vi "fpgaAcquire_exttrigtest.vi"(0 "Trigger address":i16=1500, 1 "Command FIFO":refnum<k21>, 2 "Circular Buffer Mem":refnum<k21>, 3 "circular buffer length":u32=300, 5 "Fake data in":i16, 6 "Timing FIFO":refnum<k21>, 7 "channel on/off":bool, 9 "Trigger":i16=1500, 11 "Samples to Acquire":u32=95, 12 "Is Test Pulse?":bool, 13 "# of pretrigger":u32=15, 14 "timing":u64) -> ()   [LabVIEW 2012]
uses:
  <vilib>/rvi/DataTransferAndStorage/Container/Common/niFpgaContainerExecOnDevCompGetState.vi
  <vilib>/rvi/Emulation/niFpgaSctlEmulationGetInTimedLoop.vi
  <vilib>/rvi/DataTransferAndStorage/Container/Common/niFpgaContainerGetUniqueNameForEmu.vi
  <vilib>/rvi/FIFO/Fifo_Resource/nirvififoEmulationSetSize.vi
  <vilib>/rvi/errors/niFpgaSetErrorForExecOnDevCompSimple.vi
  <vilib>/rvi/eio/common/nirviEmuReportErrorAndStop.vi
  <vilib>/rvi/Emulation/niFpgaSctlEmulationFifoFullMgr.vi
  <vilib>/rvi/Emulation/niFpgaSctlEmulationResourceMgr.vi
  <vilib>/rvi/interface/RandomDataEmulation/nirviRandomDataFPGAFIFO.vi
  <vilib>/rvi/interface/RandomDataEmulation/niFpgaRandomDataHandleErrors.vi
  <vilib>/rvi/DataTransferAndStorage/Container/XNode/niFpgaContainer.xnode
  <vilib>/rvi/FIFO/Fifo_Resource/niFpgaFifoEmulationRefIn.vi
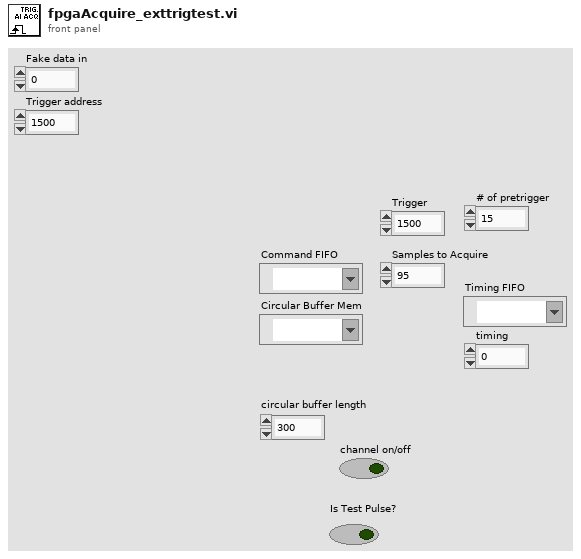
[diagram p1: front panel]
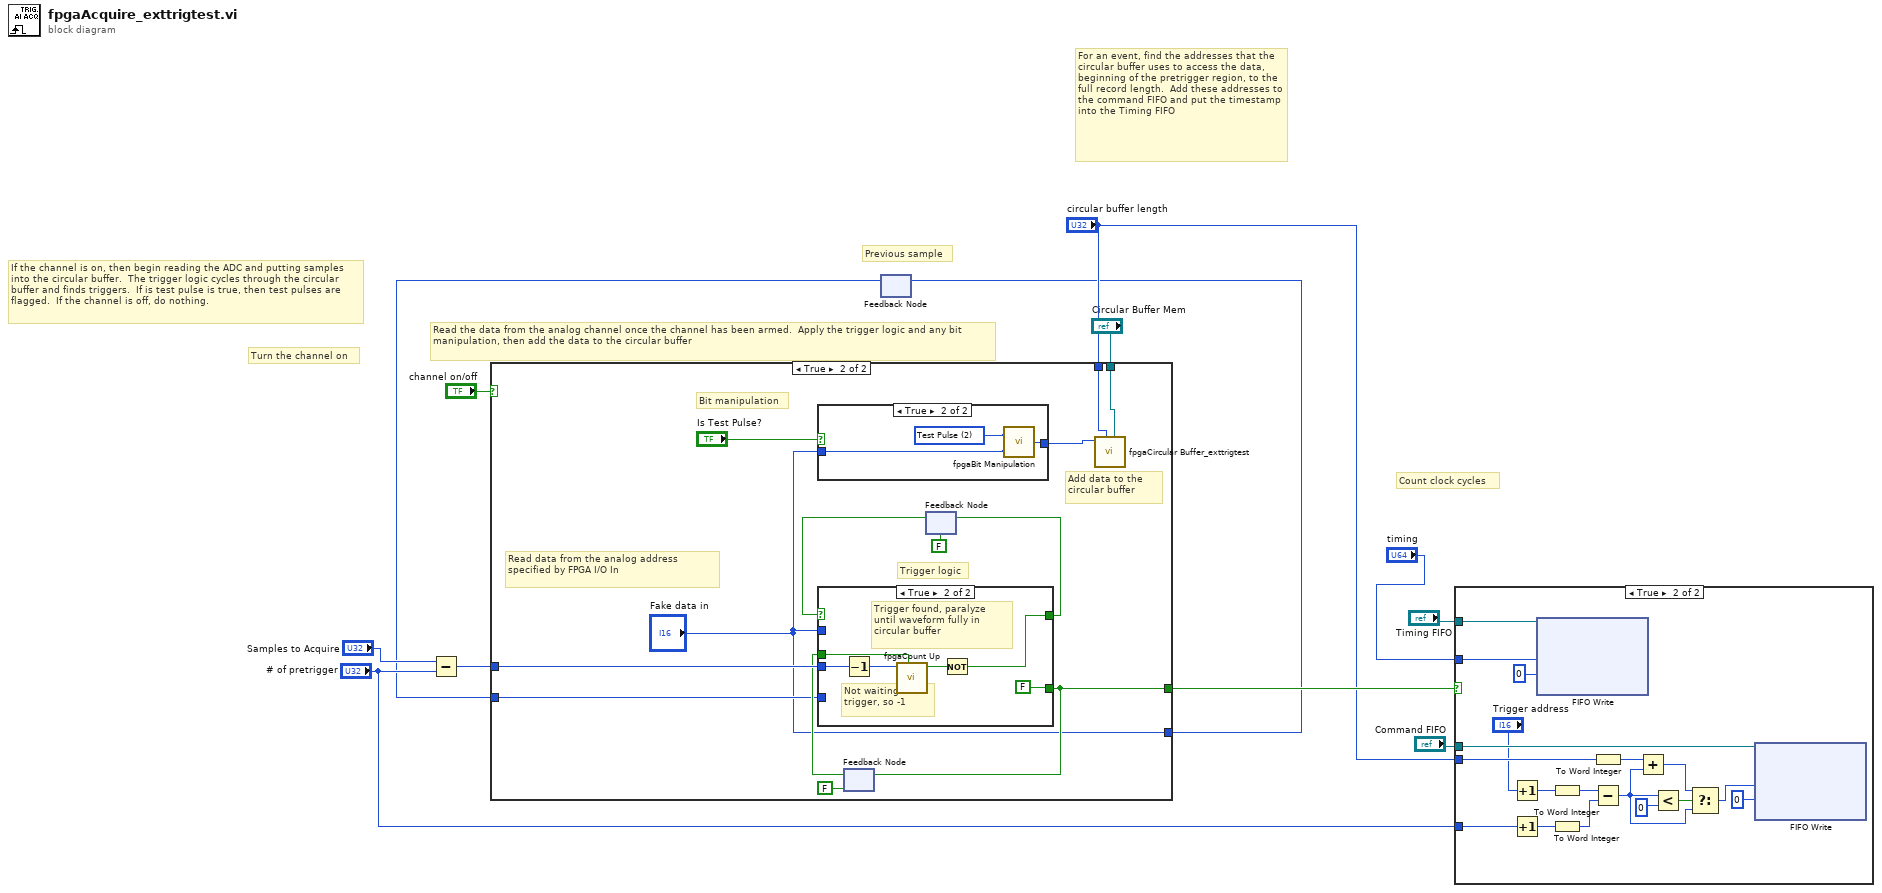
[diagram p0: block diagram]
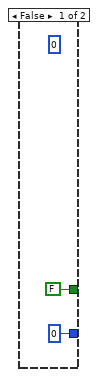
[diagram p3: hidden frame]
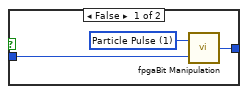
[diagram p4: hidden frame]
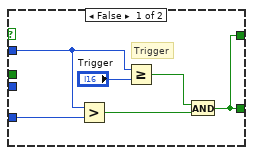
[diagram p5: hidden frame]
diagram:
  # "Previous sample"
  # "Count clock cycles"
  # "For an event, find the addresses that the circular buffer uses to access the data, beginning of the pretrigger region, to the full record length.  Add these addresses to the command FIFO and put the timestamp into the Timing FIFO"
  # "Read the data from the analog channel once the channel has been armed.  Apply the trigger logic and any bit manipulation, then add the data to the circular buffer"
  # "If the channel is on, then begin reading the ADC and putting samples into the circular buffer.  The trigger logic cycles through the circular buffer and finds triggers.  If is test pulse is true, then test pulses are flagged.  If the channel is off, do nothing."
  # "Turn the channel on"
  n1 = Subtract(x="Samples to Acquire", y="# of pretrigger") -> (x-y=w2:u32)
  n2 = feedback #1() -> (w3:i16)  [unwired: 1 in]
  n3 = case shown="True" "channel on/off" {
    tunnel: "Circular Buffer Mem" -> [_ w16]
    tunnel: "circular buffer length" -> [_ w17]
    tunnel: w2 -> [_ w25]
    tunnel: [FALSE w20] -> w12
    tunnel: [i16 0 ("Fake data in") "Fake data in"] -> w4
    tunnel: w3 -> [_ w19]
    frame False {
      (unwired) u16 0 ("Address")
    }
    frame True {
      # "Trigger logic"
      # "Read data from the analog address specified by FPGA I/O In"
      # "Add data to the circular buffer"
      # "Bit manipulation"
      n4 = case shown="True" "Is Test Pulse?" {
        tunnel: "Fake data in" -> [w29 w32]
        tunnel: [w28 w31] -> w18
        frame False {
          w30 = u16 1 items=["Header Information", "Particle Pulse", "Test Pulse"] ("Pulse Type")
          n5 = call "fpgaBit Manipulation.vi"("Pulse Type"=w30, "Integer to be written"=w29) -> ("Integer Written"=w28:i16)  [unwired: 2 in]
        }
        frame True {
          w33 = u16 2 items=["Header Information", "Particle Pulse", "Test Pulse"] ("Pulse Type")
          n6 = call "fpgaBit Manipulation.vi"("Pulse Type"=w33, "Integer to be written"=w32) -> ("Integer Written"=w31:i16)  [unwired: 2 in]
        }
      }
      n7 = feedback #2(FALSE) -> (w22:bool)
      n8 = feedback #3(FALSE) -> (w24:bool)
      n9 = case shown="True" w24 {
        tunnel: "Fake data in" -> [w36 _]
        tunnel: w25 -> [_ w41]
        tunnel: w22 -> [_ w45]
        tunnel: [w38 w43] -> w23
        tunnel: [w38 FALSE] -> w20
        tunnel: w19 -> [w34 _]
        frame False {
          # "Trigger"
          n10 = Greater?(x=w36, y=w34) -> (0:w35:bool)
          n11 = Greater Or Equal?(x=w36, y="Trigger") -> (x >= y?=w37:bool)
          n12 = And(x=w37, y=w35) -> (x .and. y?=w38:bool)
        }
        frame True {
          # "Not waiting for trigger, so -1"
          # "Trigger found, paralyze until waveform fully in circular buffer"
          n13 = Decrement(x=w41) -> (x-1=w40:u32)
          n14 = call "fpgaCount Up.vi"("Reset?"=w45, "goal"=w40) -> ("Count Met"=w44:bool)  [unwired: 8 in, 1 out]
          n15 = Not(x=w44) -> (.not. x?=w43:bool)
        }
      }
      n16 = feedback-in #2(w20) -> ()
      n17 = feedback-in #3(w23) -> ()
      n18 = call "fpgaCircular Buffer_exttrigtest.vi"("Refnum in"=w16, "Address"=w17, "Data"=w18) -> ()  [unwired: 9 in]
    }
  }
  n19 = feedback-in #1(w4) -> ()
  n20 = case shown="True" w12 {
    tunnel: "Command FIFO" -> [_ w63]
    tunnel: "Timing FIFO" -> [_ w62]
    tunnel: "circular buffer length" -> [_ w50]
    tunnel: "# of pretrigger" -> [_ w47]
    tunnel: "timing" -> [_ w49]
    frame False {
    }
    frame True {
      n21 = Increment(x="Trigger address") -> (x+1=w57:i16)
      n22 = Increment(x=w47) -> (x+1=w48:u32)
      n23 = xnode ("FIFO Write")("Element"=w49, "Timeout"=0, "FIFO In"=w62) -> ()  [unwired: 2 out]
      n24 = To Word Integer(number=w57) -> (16bit integer=w58:i16)
      n25 = To Word Integer(number=w48) -> (16bit integer=w59:i16)
      n26 = To Word Integer(number=w50) -> (16bit integer=w56:i16)
      n27 = Subtract(x=w58, y=w59) -> (x-y=w55:i16)
      n28 = Add(x=w56, y=w55) -> (x+y=w54:i16)
      n29 = Less?(x=w55, y=i16 0) -> (x < y?=w52:bool)
      n30 = Select(t=w54, s=w52, f=w55) -> (s? t:f=w51:i16)
      n31 = xnode ("FIFO Write")("Element"=w51, "Timeout"=0, "FIFO In"=w63) -> ()  [unwired: 2 out]
    }
  }
